vi "arm hold.vi"(1 "Input":dbl) -> (0 "Rate Out":dbl)   [LabVIEW 2012]
uses:
  <vilib>/addons/control/pid/pid.llb/PID (DBL).vi
  <vilib>/addons/control/pid/NI_PID_pid.lvlib
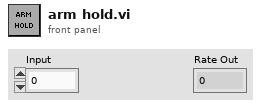
[diagram p1: front panel]
types:
  T1 = cluster{"proportional gain (Kc)":dbl, "integral time (Ti, min)":dbl, "derivative time (Td, min)":dbl}
  T2 = typedef "WPI_EncoderDevRef.ctl" = cluster{"DevStatus":errorcluster, "EncoderIndex":T3, "CounterIndex":T4, "DistancePerCount":dbl, "Decoding Type":T5}
  T3 = typedef "FPGA_EncoderIdx.ctl" = enum8{"Enc 0", "Enc 1", "Enc 2", "Enc 3", "Invalid"}
  T4 = typedef "FPGA_CounterCtrSystemIndex.ctl" = enum8{"Ctr 0", "Ctr 1", "Ctr 2", "Ctr 3", "Ctr 4", "Ctr 5", "Ctr 6", "Ctr 7", "Invalid"}
  T5 = typedef "WPI_EncoderType.ctl" = enum16{"1x", "2x", "4x"}
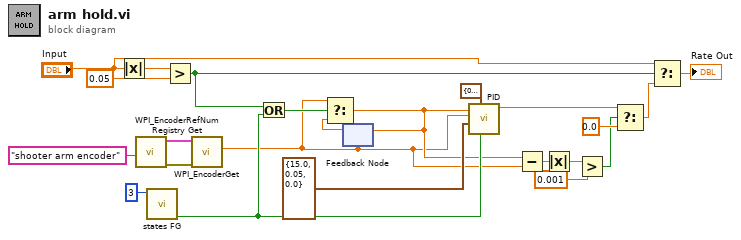
[diagram p0: block diagram]
diagram:
  n1 = Absolute Value(x="Input") -> (abs(x)=w11:dbl)
  n2 = call <vilib>:"WPI_EncoderRefNum Registry Get.vi"("refnum name"="shooter arm encoder") -> ("error out"=w18:errorcluster, "EncoderDevRef"=w17:T2)  [unwired: 9 in]
  n3 = call "states FG.vi"("Loop ID"=3) -> ("first call?"=w14:bool)  [unwired: 7 in, 3 out]
  n4 = Greater?(x=w11, y=0.05) -> (0:w10:bool)
  n5 = call <vilib>:"WPI_EncoderGet.vi"("error in (no error)"=w18, "EncoderDevRef"=w17) -> ("Distance"=w8:dbl)  [unwired: 4 in, 5 out]
  n6 = Or(x=w10, y=w14) -> (x .or. y?=w13:bool)
  n7 = feedback #1(w8) -> (w12:dbl)
  n8 = Select(t=w8, s=w13, f=w12) -> (s? t:f=w9:dbl)
  n9 = feedback-in #1(w9) -> ()
  n10 = call-poly <vilib>:"PID.vi"("reinitialize? (F)"=w14, "output range"=cluster{"output high":dbl, "output low":dbl} {"output high"=0.25, "output low"=-0.25}, "PID gains"=T1 {"proportional gain (Kc)"=15.0, "integral time (Ti, min)"=0.05, "derivative time (Td, min)"=0.0}, "process variable"=w8, "setpoint"=w9) -> ("output"=w5:dbl)  [unwired: 5 in, 1 out]
  n11 = Subtract(x=w9, y=w8) -> (x-y=w7:dbl)
  n12 = Absolute Value(x=w7) -> (abs(x)=w3:dbl)
  n13 = Greater?(x=w3, y=0.001) -> (0:w1:bool)
  n14 = Select(t=w5, s=w1, f=0.0) -> (s? t:f=w6:dbl)
  n15 = Select(t="Input", s=w10, f=w6) -> (s? t:f=→"Rate Out":dbl)
